vi "terminate.vi"(8 "error in (no error)":errorcluster, 11 "MG090622IMAQCamera in":refnum<class "DAQ_MG090622Camera.lvclass">) -> (0 "error out":errorcluster, 3 "MG090622IMAQCamera out":refnum<class "DAQ_MG090622Camera.lvclass">)   [LabVIEW 2010, in "DAQ_MG090622Camera.lvclass"]
doc: "The dynamic dispatch version of this VI terminates the plug-in object by releasing all of its resources."
uses:
  DAQ_MG090622Camera.lvclass
  <vilib>/userDefined/High Color/IMAQdx.ctl
  DAQ_MG090622Camera.lvclass/DAQ_MG090622Camera.ctl
  common/classes/Image/Image/Image.lvclass
  DAQ_DL090211Scaffold/DAQ_DL090211Scaffold/DAQ_DL090211Scaffold.lvclass
  common/classes/ErrorController/ErrorController/class_data.vi
  common/classes/ErrorController/ErrorController/ErrorController.lvclass
  <vilib>/vision/driver/NI_Vision_Acquisition_Software.lvlib
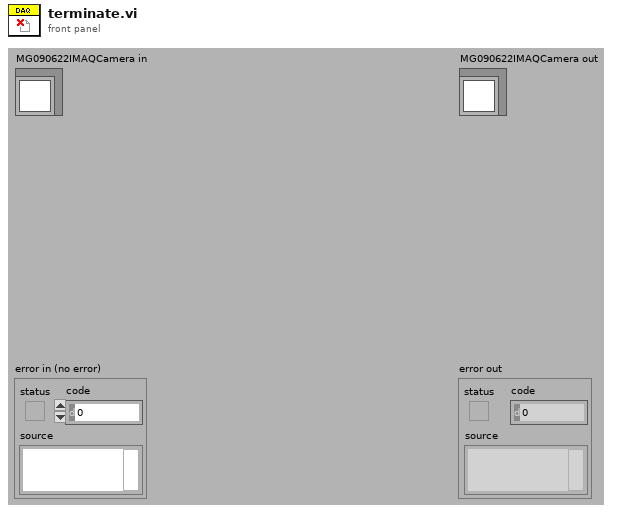
[diagram p1: front panel]
types:
  T1 = typedef "IMAQdx.ctl" = refnum<k21>
  T2 = typedef "DAQ_MG090622Camera.lvclass/connection_type_enum.ctl" = enum16{"IEEE 1394 (FireWire)", "USB", "GigE", "CameraLink"}
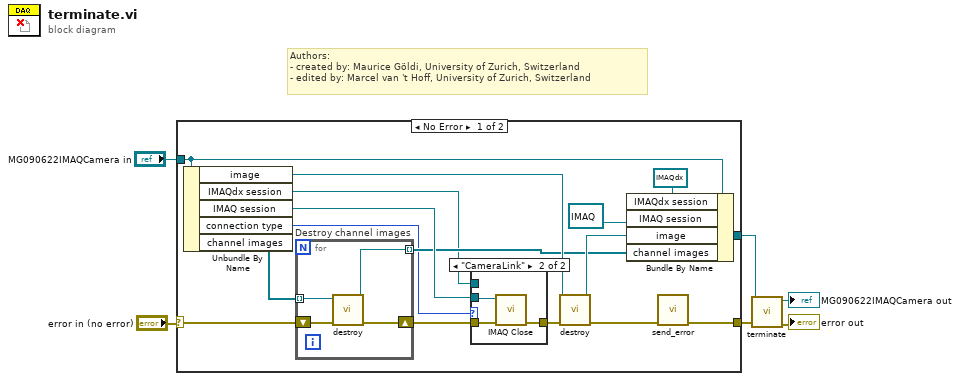
[diagram p0: block diagram]
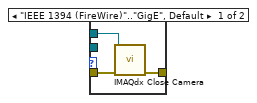
[diagram p2: hidden frame]
diagram:
  # "Authors: \n- created by: Maurice Göldi, University of Zurich, Switzerland\n- edited by: Marcel van 't Hoff, University of Zurich, Switzerland"
  n1 = case shown="No Error" "error in (no error)" {
    selector: "error in (no error)" -> [w16 w34]
    tunnel: [w11 w34] -> w3
    tunnel: [w21 w33] -> w1
    tunnel: "MG090622IMAQCamera in" -> [w20 w33]
    frame No Error {
      n2 = Unbundle By Name(w20) -> ("image"=w18:refnum<class "Image.lvclass">, "IMAQdx session"=w8:T1, "IMAQ session"=w22:refnum<k11>, "connection type"=w9:T2, "channel images"=w10:refnum<class "Image.lvclass">[])
      n3 = for "Destroy channel images" {
        shift-right: [w32] -> w15
        shift-left: w16 -> [w30]
        tunnel: w10 -> [w29] mode=indexing
        tunnel: [w31] -> w14 mode=indexing
        n4 = call-dynamic "destroy.vi"("error in (no error)"=w30, "Image in"=w29) -> ("error out"=w32:errorcluster, "Image out"=w31:refnum<class "Image.lvclass">)  [unwired: 8 out]
      }
      n5 = case shown="\"CameraLink\"" w9 {
        tunnel: w22 -> [_ w26]
        tunnel: [w24 w27] -> w19
        tunnel: w15 -> [w25 w28]
        tunnel: w8 -> [w23 _]
        frame "IEEE 1394 (FireWire)".."GigE", Default {
          n6 = call <vilib>:"IMAQdx Close Camera.vi"("error in"=w25, "Session In"=w23) -> ("error out"=w24:errorcluster)  [unwired: 9 in]
        }
        frame "CameraLink" {
          n7 = call <vilib>:"IMAQ Close.vi"("error in (no error)"=w28, "IMAQ Session In"=w26) -> ("error out"=w27:errorcluster)  [unwired: 9 out]
        }
      }
      n8 = call-dynamic "destroy.vi"("error in (no error)"=w19, "Image in"=w18) -> ("error out"=w12:errorcluster, "Image out"=w17:refnum<class "Image.lvclass">)  [unwired: 8 out]
      n9 = Bundle By Name(cluster=w20, "IMAQdx session"=T1 refnum, "IMAQ session"=refnum<k11> refnum ("IMAQ Session"), "image"=w17, "channel images"=w14) -> (w21:refnum<class "DAQ_MG090622Camera.lvclass">)
      n10 = call "send_error.vi"("error in (no error)"=w12) -> ("error out"=w11:errorcluster)  [unwired: 10 in]
    }
    frame Error {
    }
  }
  n11 = call-parent "terminate.vi"("error in (no error)"=w3, "GenericPlugin in"=w1) -> ("error out"=→"error out":errorcluster, "GenericPlugin out"=→"MG090622IMAQCamera out":refnum<class "DAQ_MG090622Camera.lvclass">)  [unwired: 8 out]
